vi "Autonomous Independent.vi"   [LabVIEW 2012]
doc: "This VI is called when autonomous begins, and will automatically be terminated when autonomous ends. You can carry out timed or sensor driven robot movement independently without needing to return to the caller."
uses:
  <vilib>/Rock Robotics/WPI/Relay/WPI_RelayValue.ctl
  Robot Global Data.vi
types:
  T1 = typedef "WPI_EncoderDevRef.ctl" = cluster{"DevStatus":errorcluster, "EncoderIndex":T2, "CounterIndex":T3, "DistancePerCount":dbl, "Decoding Type":T4}
  T2 = typedef "FPGA_EncoderIdx.ctl" = enum8{"Enc 0", "Enc 1", "Enc 2", "Enc 3", "Invalid"}
  T3 = typedef "FPGA_CounterCtrSystemIndex.ctl" = enum8{"Ctr 0", "Ctr 1", "Ctr 2", "Ctr 3", "Ctr 4", "Ctr 5", "Ctr 6", "Ctr 7", "Invalid"}
  T4 = typedef "WPI_EncoderType.ctl" = enum16{"1x", "2x", "4x"}
  T5 = typedef "WPI_GyroDevRef.ctl" = cluster{"DevStatus":errorcluster, "Analog Module":T6, "Analog Channel":T7, "Offset":dbl, "Gain (VoltsPerDegree/Second)":dbl}
  T6 = typedef "FPGA_TypedefAnalogModule.ctl" = enum16{"Analog Module 1", "Analog Module 2"}
  T7 = typedef "FPGA_AIChannel.ctl" = enum8{"AI 1", "AI 2", "AI 3", "AI 4", "AI 5", "AI 6", "AI 7", "AI 8", "Invalid"}
  T8 = typedef "WPI_MotorControlDeviceRef.ctl" = cluster{"DeviceStatus":errorcluster, "Type":enum16{"PWM", "CAN"}, "PWM":cluster{"Digital Module":T9, "PWM Channel":T10, "DeadBand":T11}, "CAN":cluster{"Device Number":u8, "Control Mode":T12, "Semaphore":T13, "Max Vout":dbl}, "Invert":bool, "TransformRef":T14, "InvTransformRef":T14}
  T9 = typedef "FPGA_TypedefDigitalModule.ctl" = enum16{"Digital Module 1", "Digital Module 2"}
  T10 = typedef "FPGA_DIOPWMChannel.ctl" = enum8{"PWM 1", "PWM 2", "PWM 3", "PWM 4", "PWM 5", "PWM 6", "PWM 7", "PWM 8", "PWM 9", "PWM 10", "Invalid"}
  T11 = typedef "WPI_PWMDeadband.ctl" = cluster{"Name":string, "maxPositivePwm":i32, "minPositivePwm":i32, "centerPwm":i32, "maxNegativePwm":i32, "minNegativePwm":i32, "angularRange":u16}
  T12 = typedef "WPI_CANJaguar_ControlMode.ctl" = enum8{"Percent VBus", "Current", "Speed", "Position", "Voltage"}
  T13 = typedef "Semaphore RefNum" = refnum<k1>
  T14 = typedef "WPI_PWMTransform_ConPane.ctl" = refnum<vi>
  T15 = typedef "WPI_DigitalInputDevRef.ctl" = cluster{"DevStatus":errorcluster, "DIO Channel":T16, "Digital Module":T9}
  T16 = typedef "FPGA_DIOChannel.ctl" = enum8{"DIO 1", "DIO 2", "DIO 3", "DIO 4", "DIO 5", "DIO 6", "DIO 7", "DIO 8", "DIO 9", "DIO 10", "DIO 11", "DIO 12", "DIO 13", "DIO 14", "Invalid"}
  T17 = typedef "WPI_RelayValue.ctl" = enum16{"Off", "On", "Forward", "Reverse"}
  T18 = cluster{"Shifting":cluster{"Right Servo High":dbl, "Right Servo Low":dbl, "Left Servo High":dbl, "Left Servo Low":dbl}, "Breaking":cluster{"Coast Position":dbl, "Break Position":dbl}}
  T19 = cluster{"Right Servo High":dbl, "Right Servo Low":dbl, "Left Servo High":dbl, "Left Servo Low":dbl}
  T20 = typedef "WPI_RelayDevRef.ctl" = cluster{"DevStatus":errorcluster, "Relay Channel":T21, "Digital Module":T9, "Relay Direction":T22}
  T21 = typedef "FPGA_DIORelayChannel.ctl" = enum8{"Relay 1", "Relay 2", "Relay 3", "Relay 4", "Relay 5", "Relay 6", "Relay 7", "Relay 8", "Invalid"}
  T22 = typedef "WPI_RelayDirection.ctl" = enum16{"Both directions", "Forward only", "Reverse only"}
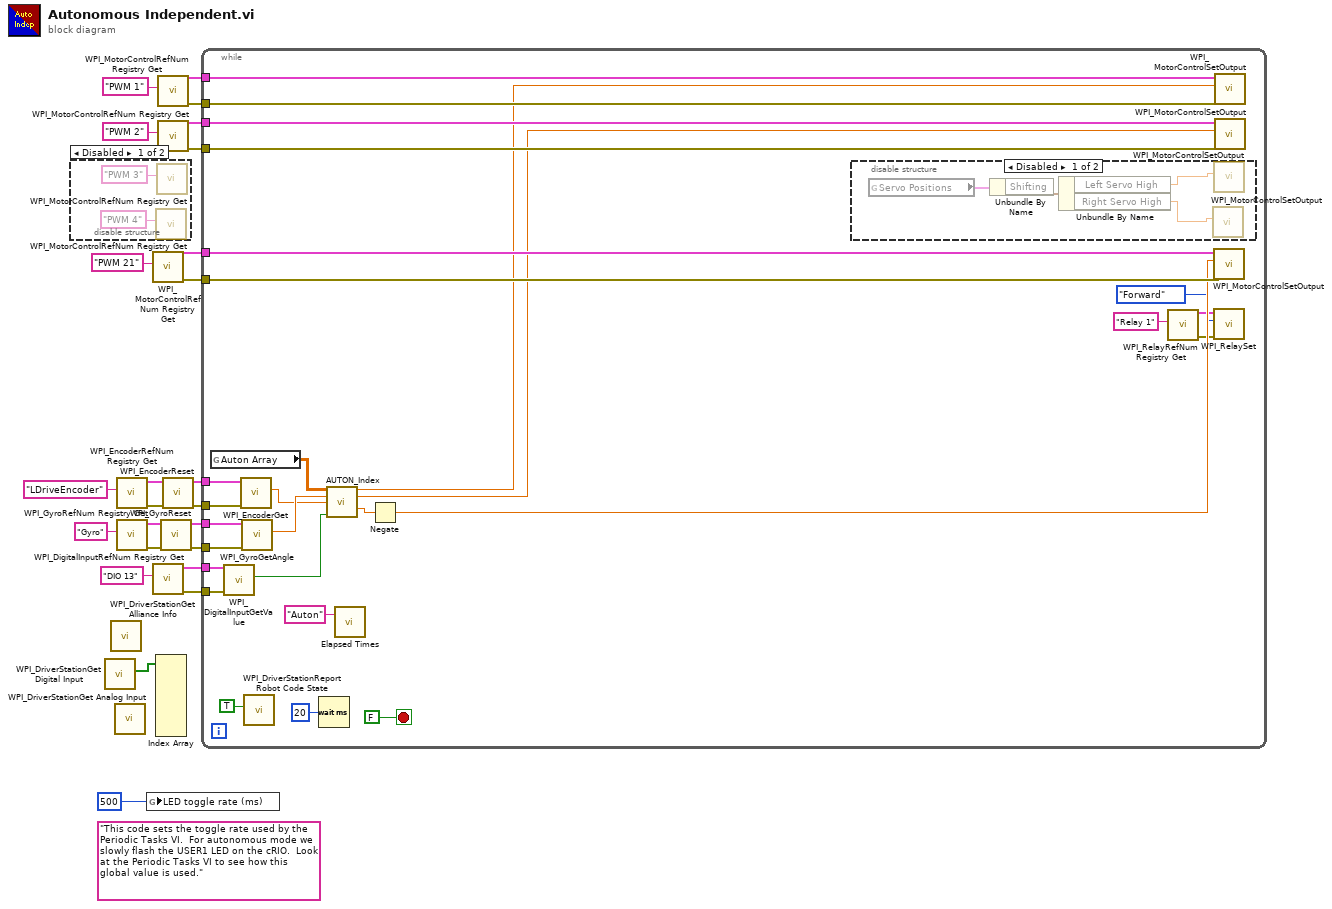
[diagram p0: block diagram]
diagram:
  (unwired) "This code sets the toggle rate used by the Periodic Tasks VI.  For autonomous mode we slowly flash the USER1 LED on the cRIO.  Look at the Periodic Tasks VI to see how this global value is used."
  n1 = disable-structure shown="Disabled" {
    frame Disabled {
      n2 = call <vilib>:"WPI_MotorControlRefNum Registry Get.vi"("refnum name"="PWM 4") -> ()  [unwired: 9 in, 2 out]
      n3 = call <vilib>:"WPI_MotorControlRefNum Registry Get.vi"("refnum name"="PWM 3") -> ()  [unwired: 9 in, 2 out]
    }
    frame Enabled {
    }
  }
  n4 = call <vilib>:"WPI_DriverStationGet Digital Input.vi"() -> ("Driver Station Digital Input (1-8)"=w24:bool[])  [unwired: 11 out]
  n5 = call <vilib>:"WPI_DriverStationGet Alliance Info.vi"() -> ()  [unwired: 12 out]
  n6 = call <vilib>:"WPI_DriverStationGet Analog Input.vi"() -> ()  [unwired: 12 out]
  n7 = call <vilib>:"WPI_EncoderRefNum Registry Get.vi"("refnum name"="LDriveEncoder") -> ("error out"=w7:errorcluster, "EncoderDevRef"=w6:T1)  [unwired: 9 in]
  n8 = call <vilib>:"WPI_GyroRefNum Registry Get.vi"("refnum name"="Gyro") -> ("error out"=w11:errorcluster, "GyroDevRef"=w12:T5)  [unwired: 9 in]
  n9 = global write "Robot Global Data.vi" "LED toggle rate (ms)"(u32 500 ("LED ms toggle rate")) -> ()
  n10 = call <vilib>:"WPI_MotorControlRefNum Registry Get.vi"("refnum name"="PWM 21") -> ("error out"=w14:errorcluster, "MotorControlDevRef"=w15:T8)  [unwired: 9 in]
  n11 = call <vilib>:"WPI_DigitalInputRefNum Registry Get.vi"("refnum name"="DIO 13") -> ("error out"=w2:errorcluster, "DigitalInputDevRef"=w3:T15)  [unwired: 9 in]
  n12 = Index Array(array=w24) -> ()  [unwired: 8 in, 8 out]
  n13 = call <vilib>:"WPI_MotorControlRefNum Registry Get.vi"("refnum name"="PWM 1") -> ("error out"=w20:errorcluster, "MotorControlDevRef"=w21:T8)  [unwired: 9 in]
  n14 = call <vilib>:"WPI_MotorControlRefNum Registry Get.vi"("refnum name"="PWM 2") -> ("error out"=w19:errorcluster, "MotorControlDevRef"=w18:T8)  [unwired: 9 in]
  n15 = call <vilib>:"WPI_GyroReset.vi"("error in (no error)"=w11, "GyroDevRef"=w12) -> ("error out"=w9:errorcluster, "GyroDevRef"=w10:T5)  [unwired: 8 in]
  n16 = call <vilib>:"WPI_EncoderReset.vi"("error in (no error)"=w7, "EncoderDevRef"=w6) -> ("error out"=w4:errorcluster, "EncoderDevRef"=w5:T1)  [unwired: 8 in]
  n17 = while {
    tunnel: w21 -> [w51]
    tunnel: w20 -> [w50]
    tunnel: w18 -> [w48]
    tunnel: w19 -> [w49]
    tunnel: w15 -> [w45]
    tunnel: w14 -> [w44]
    tunnel: w10 -> [w39]
    tunnel: w9 -> [w38]
    tunnel: w5 -> [w37]
    tunnel: w4 -> [w36]
    tunnel: w3 -> [w28]
    tunnel: w2 -> [w29]
    stop <- FALSE stop-if-true
    n18 = global read "Robot Global Data.vi" "Auton Array"() -> (w47:dbl[][])
    n19 = call <vilib>:"WPI_DigitalInputGetValue.vi"("error in (no error)"=w29, "DigitalInputDevRef"=w28) -> ("Value"=w27:bool)  [unwired: 7 in, 2 out]
    n20 = call <vilib>:"WPI_EncoderGet.vi"("error in (no error)"=w36, "EncoderDevRef"=w37) -> ("Distance"=w35:dbl)  [unwired: 4 in, 5 out]
    n21 = call <vilib>:"WPI_GyroGetAngle.vi"("error in (no error)"=w38, "GyroDevRef"=w39) -> ("Angle"=w46:dbl)  [unwired: 6 in, 3 out]
    n22 = call <vilib>:"WPI_DriverStationReport Robot Code State.vi"("Autonomous"=TRUE) -> ()  [unwired: 10 in, 1 out]
    n23 = Wait (ms)(milliseconds to wait=u32 20) -> ()  [unwired: 1 out]
    n24 = call "AUTON_Index.vi"("Auton Array"=w47, "MeasuredHeading"=w46, "LeftEncoder"=w35, "Harvester DIO"=w27) -> ("Left Drive"=w40:dbl, "Right Drive"=w41:dbl, "Shooter Elevation"=w43:dbl)  [unwired: 5 in, 4 out]
    n25 = call "Elapsed Times.vi"("Call Name"="Auton") -> ()  [unwired: 2 in, 1 out]
    n26 = Negate(x=w43) -> (-x=w42:dbl)
    n27 = disable-structure shown="Disabled" {
      frame Disabled {
        n28 = global read "Robot Global Data.vi" "Servo Positions"() -> (w58:T18)
        n29 = Unbundle By Name(w58) -> ("Shifting"=w57:T19)
        n30 = Unbundle By Name(w57) -> ("Left Servo High"=w56:dbl, "Right Servo High"=w55:dbl)
        n31 = call <vilib>:"WPI_MotorControlSetOutput.vi"("Output"=w55) -> ()  [unwired: 8 in, 3 out]
        n32 = call <vilib>:"WPI_MotorControlSetOutput.vi"("Output"=w56) -> ()  [unwired: 8 in, 3 out]
      }
      frame Enabled {
      }
    }
    n33 = call <vilib>:"WPI_RelayRefNum Registry Get.vi"("refnum name"="Relay 1") -> ("error out"=w31:errorcluster, "RelayDevRef"=w33:T20)  [unwired: 9 in]
    n34 = call <vilib>:"WPI_MotorControlSetOutput.vi"("error in (no error)"=w44, "Output"=w42, "MotorControlDevRef"=w45) -> ()  [unwired: 6 in, 3 out]
    n35 = call <vilib>:"WPI_RelaySet.vi"("error in (no error)"=w31, "RelayValue"=WPI_RelayValue."Forward", "RelayDevRef"=w33) -> ()  [unwired: 7 in, 2 out]
    n36 = call <vilib>:"WPI_MotorControlSetOutput.vi"("error in (no error)"=w50, "Output"=w40, "MotorControlDevRef"=w51) -> ()  [unwired: 6 in, 3 out]
    n37 = call <vilib>:"WPI_MotorControlSetOutput.vi"("error in (no error)"=w49, "Output"=w41, "MotorControlDevRef"=w48) -> ()  [unwired: 6 in, 3 out]
  }
